vi "curl commands.vi"() -> ()   [LabVIEW 2019]
panel:
  in  "Request":enum16{"TOKEN", "STATUS", "RELOAD"}(ring)
  out "resulting string":string
  in  "Secret":string
  in  "Token":string
  in  "Address":string
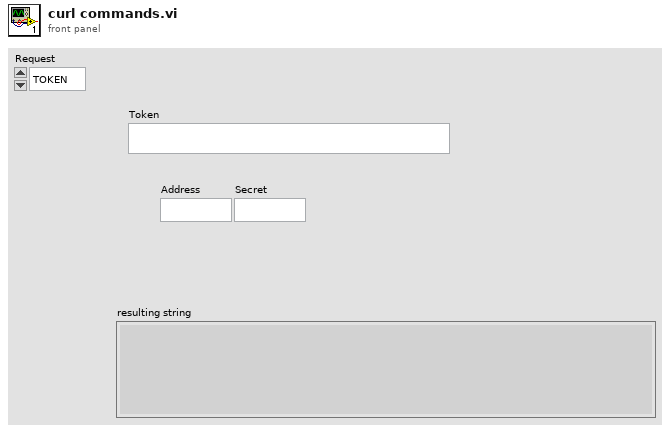
[diagram p1: front panel]
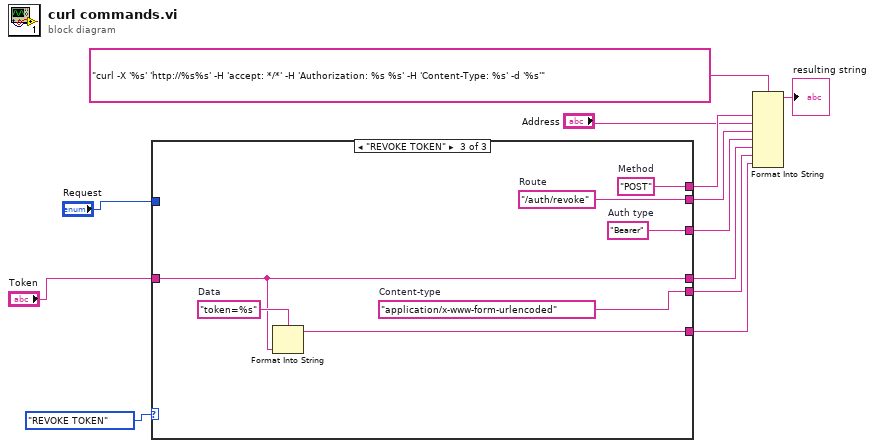
[diagram p0: block diagram]
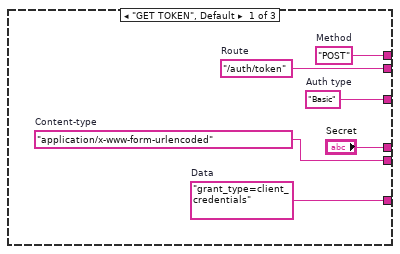
[diagram p2: hidden frame]
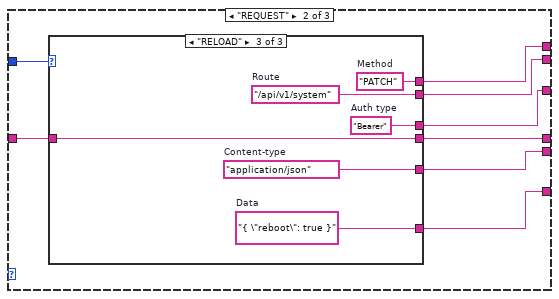
[diagram p3: hidden frame]
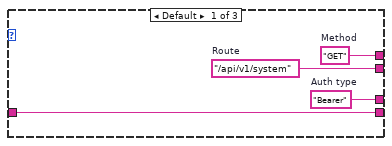
[diagram p4: hidden frame]
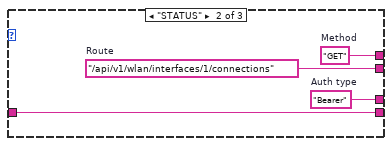
[diagram p5: hidden frame]
diagram:
  n1 = case shown="\"REVOKE TOKEN\"" enum16{"GET TOKEN", "REQUEST", "REVOKE TOKEN"}."REVOKE TOKEN" ("States") {
    tunnel: [w18 w26 w47] -> w12
    tunnel: [w17 w25 w46] -> w11
    tunnel: [w16 w24 w45] -> w10
    tunnel: ["Secret" w19 w41] -> w9
    tunnel: [w14 w22 w44] -> w8
    tunnel: [w13 w21 w42] -> w7
    tunnel: "Token" -> [_ w23 w41]
    tunnel: "Request" -> [_ w20 _]
    frame "GET TOKEN", Default {
      w13 = "grant_type=client_credentials"  # Data
      w14 = "application/x-www-form-urlencoded"  # Content-type
      w16 = "Basic"  # Auth type
      w17 = "/auth/token"  # Route
      w18 = "POST"  # Method
    }
    frame "REQUEST" {
      n2 = case shown="\"RELOAD\"" w20 {
        tunnel: [w30 w34 w40] -> w26
        tunnel: [w29 w33 w39] -> w25
        tunnel: [w28 w32 w38] -> w24
        tunnel: w23 -> [w27 w31 w37]
        tunnel: [w27 w31 w37] -> w19
        tunnel: [_ _ w36] -> w22
        tunnel: [_ _ w35] -> w21
        frame Default {
          w28 = "Bearer"  # Auth type
          w29 = "/api/v1/system"  # Route
          w30 = "GET"  # Method
        }
        frame "STATUS" {
          w32 = "Bearer"  # Auth type
          w33 = "/api/v1/wlan/interfaces/1/connections"  # Route
          w34 = "GET"  # Method
        }
        frame "RELOAD" {
          w35 = "{ \"reboot\": true }"  # Data
          w36 = "application/json"  # Content-type
          w38 = "Bearer"  # Auth type
          w39 = "/api/v1/system"  # Route
          w40 = "PATCH"  # Method
        }
      }
    }
    frame "REVOKE TOKEN" {
      w43 = "token=%s"  # Data
      w44 = "application/x-www-form-urlencoded"  # Content-type
      w45 = "Bearer"  # Auth type
      w46 = "/auth/revoke"  # Route
      w47 = "POST"  # Method
      n3 = Format Into String(format string=w43, w41) -> (resulting string=w42:string)  [unwired: 2 in, 1 out]
    }
  }
  n4 = Format Into String(format string="curl -X '%s' 'http://%s%s' -H 'accept: */*' -H 'Authorization: %s %s' -H 'Content-Type: %s' -d '%s'", w12, "Address", w11, w10, w9, w8, w7) -> (resulting string=→"resulting string":string)  [unwired: 2 in, 1 out]
